vi "sample.vi"() -> ()   [LabVIEW 2012]
panel:
  out "Option Read":string
  out "Data":string
  out "Address":string
  in  "Option Write":enum16{"Off", "Once", "Continuous", "Stop"}(ring)
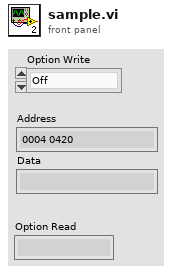
[diagram p1: front panel]
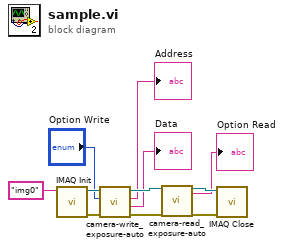
[diagram p0: block diagram]
diagram:
  n1 = call <vilib>:"IMAQ Init.vi"("Interface Name"="img0") -> ("error out"=w8:errorcluster, "IMAQ Session Out"=w9:refnum<k11>)  [unwired: 9 in]
  n2 = call "camera-write_exposure-auto.vi"("error in (no error)"=w8, "Option"="Option Write", "IMAQ Session In"=w9) -> ("error out"=w7:errorcluster, "Data"=→"Data":string, "Address"=→"Address":string, "IMAQ Session Out"=w11:refnum<k11>)  [unwired: 3 in]
  n3 = call "camera-read_exposure-auto.vi"("IMAQ Session In"=w11, "error in (no error)"=w7) -> ("IMAQ Session Out"=w3:refnum<k11>, "Option"=→"Option Read":string, "error out"=w1:errorcluster)  [unwired: 13 in, 2 out]
  n4 = call <vilib>:"IMAQ Close.vi"("error in (no error)"=w1, "IMAQ Session In"=w3) -> ()  [unwired: 9 in, 1 out]
